vi "CreateDouble.vi"(4 "Numeric 3":u8, 5 "Numeric 9":u8, 6 "Numeric 4":u8, 7 "Numeric 8":u8, 8 "Numeric 5":u8, 9 "Numeric 6":u8, 10 "Numeric in":u8, 11 "Numeric 7":u8) -> (3 "Numeric out":dbl)   [LabVIEW 2015]
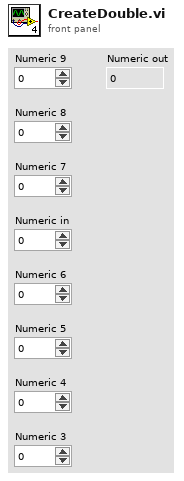
[diagram p1: front panel]
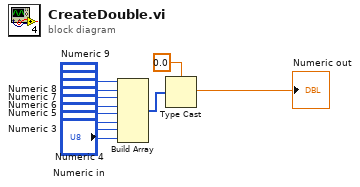
[diagram p0: block diagram]
diagram:
  w10 = 0.0
  n1 = Build Array("Numeric 9", "Numeric 8", "Numeric 7", "Numeric 6", "Numeric 5", "Numeric 4", "Numeric 3", "Numeric in") -> (w9:u8[])
  n2 = Type Cast(type=w10, x=w9) -> ()  [unwired: 1 out]
  "Numeric out" <- w10
